vi "simple calculator.vi"(8 "Y":dbl, 9 "X":dbl) -> (0 "X/Y":dbl, 1 "X*Y":dbl, 2 "X-Y":dbl, 3 "X+Y":dbl)   [LabVIEW 2016]
panel:
  in  "stop":bool
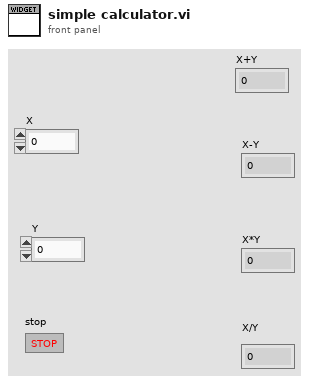
[diagram p1: front panel]
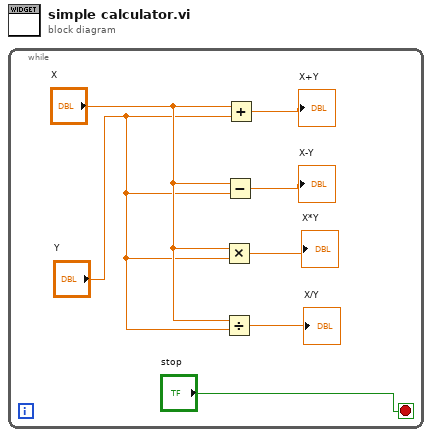
[diagram p0: block diagram]
diagram:
  n1 = while {
    stop <- "stop" stop-if-true
    n2 = Multiply(x="X", y="Y") -> (x*y=→"X*Y":dbl)
    n3 = Divide(x="X", y="Y") -> (x/y=→"X/Y":dbl)
    n4 = Subtract(x="X", y="Y") -> (x-y=→"X-Y":dbl)
    n5 = Add(x="X", y="Y") -> (x+y=→"X+Y":dbl)
  }
